vi "piezoSawtoothWave.vi"(0 "dt":dbl=0.00019996 format="%#_13g", 1 "nT":i32=1667, 2 "t0":dbl, 3 "omega":dbl=9.42478, 4 "amplitude":dbl=1.0, 5 "smoothing param":dbl=0.001 format="%#_13g", 8 "offset":dbl=5.0 format="%#_13g") -> (7 "x+y":dbl[](array[numeric]))   [LabVIEW 2017]
uses:
  <vilib>/measure/NI_MAPro.lvlib
  <vilib>/measure/maspectr.llb/FFT Power Spectrum and PSD for 1 Chan.vi
panel:
  out "Spectrum":cluster{"f0":dbl, "df":dbl, "magnitude":dbl[]}(graph)
  out "Waveform Graph":dbl[](graph)
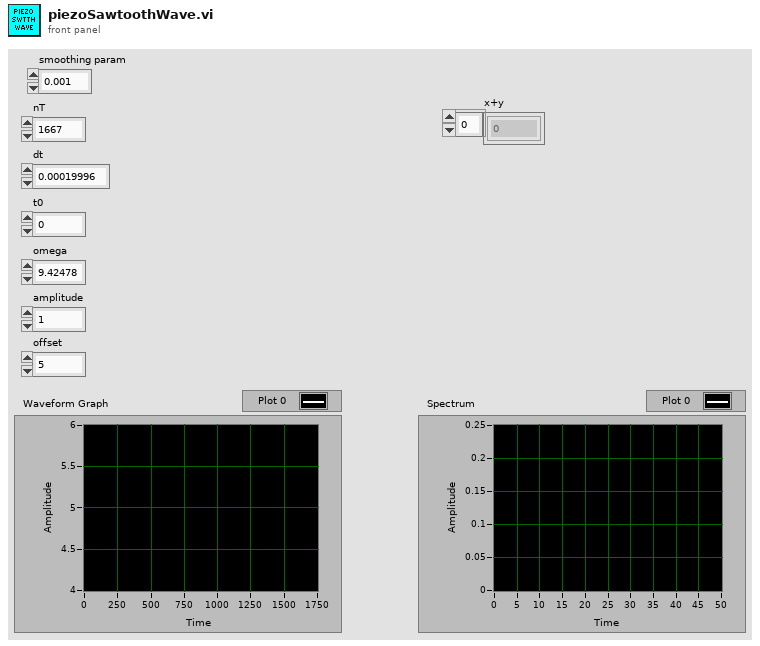
[diagram p1: front panel]
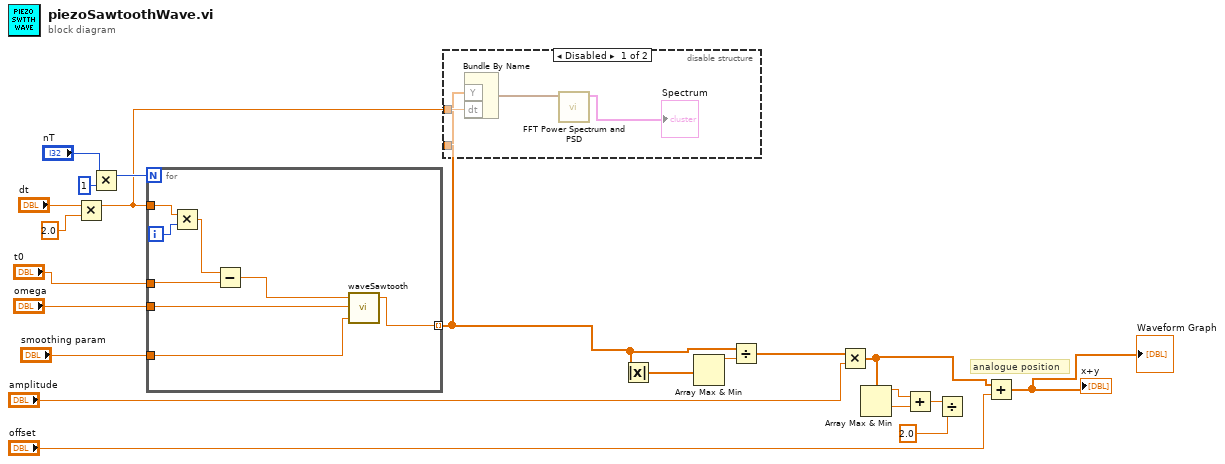
[diagram p0: block diagram]
diagram:
  # "analogue position"
  n1 = Multiply(x="dt", y=2.0) -> (x*y=w3:dbl)
  n2 = Multiply(x="nT", y=1) -> (x*y=w5:i32)
  n3 = for {
    N: w5 -> [_]
    tunnel: w3 -> [w29]
    tunnel: "omega" -> [w27]
    tunnel: "t0" -> [w26]
    tunnel: [w22] -> w2 mode=indexing
    tunnel: "smoothing param" -> [w23]
    i -> [w28]
    n4 = Multiply(x=w29, y=w28) -> (x*y=w25:dbl)
    n5 = Subtract(x=w25, y=w26) -> (x-y=w24:dbl)
    n6 = call "waveSawtooth.vi"("smoothing param"=w23, "w"=w27, "t"=w24) -> ("sawtooth"=w22:dbl)  [unwired: 2 out]
  }
  n7 = disable-structure shown="Disabled" {
    disable-tunnel: w3 -> [w33 _]
    disable-tunnel: w2 -> [w32 _]
    frame Disabled {
      n8 = Bundle By Name("Y"=w32, "dt"=w33) -> (w31:waveform(dbl))  [unwired: 1 in]
      n9 = call-poly <vilib>:"FFT Power Spectrum and PSD.vi"("time signal"=w31) -> ("Power Spectrum / PSD"=→"Spectrum":cluster{"f0":dbl, "df":dbl, "magnitude":dbl[]})  [unwired: 7 in, 3 out]
    }
    frame Enabled {
    }
  }
  n10 = Absolute Value(x=w2) -> (abs(x)=w13:dbl[])
  n11 = Array Max & Min(array=w13) -> (max value=w12:dbl)  [unwired: 3 out]
  n12 = Divide(x=w2, y=w12) -> (x/y=w9:dbl[])
  n13 = Multiply(x=w9, y="amplitude") -> (x*y=w10:dbl[])
  n14 = Array Max & Min(array=w10) -> (max value=w19:dbl, min value=w18:dbl)  [unwired: 2 out]
  n15 = Add(x=w19, y=w18) -> (x+y=w17:dbl)
  n16 = Divide(x=w17, y=2.0) -> ()  [unwired: 1 out]
  n17 = Add(x=w10, y="offset") -> (x+y=→"x+y" →"Waveform Graph":dbl[])
